vi "Save_Raw_data.vi"(4 "Add to Block Header":string, 5 "PWA Binary":i16[][](array[numeric]), 6 "Analogue Binary":i16[][](array[numeric]), 7 "append to file? (new file:F)":bool, 8 "Block Timings":T1={"Started"=0.0, "Ended"=0.0, "Analogue Frequency Hz"=1000.0} {"Analogue Frequency Hz" format="%.2f"}, 9 "LDA Binary":u16[][](array[numeric])) -> (2 "Block Header":string)   [LabVIEW 2011]
uses:
  Controls/Block_start_and_end.ctl
  Globals/LDA_meas_global_1.vi
  Globals/Constants_global.vi
  Globals/LDA_meas_global_2.vi
  Globals/Meas_global.vi
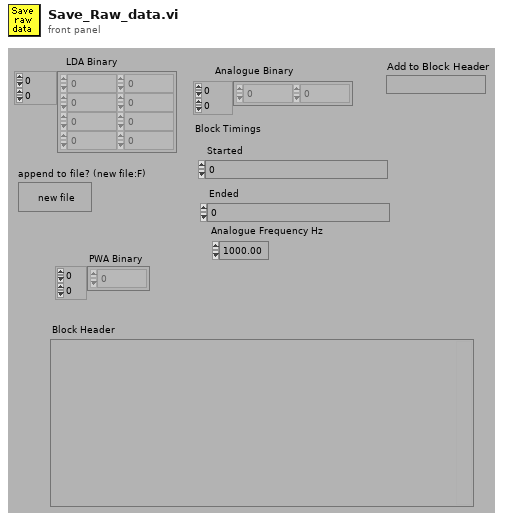
[diagram p1: front panel]
types:
  T1 = typedef "Block_start_and_end.ctl" = cluster{"Started":dbl, "Ended":dbl, "Analogue Frequency Hz":dbl}
  T2 = cluster{"scale multiplier":dbl, "scale offset":dbl}[]
  T3 = typedef "PWA_Data.ctl" = enum16{"No PWA Data", "One Ch PWA"}
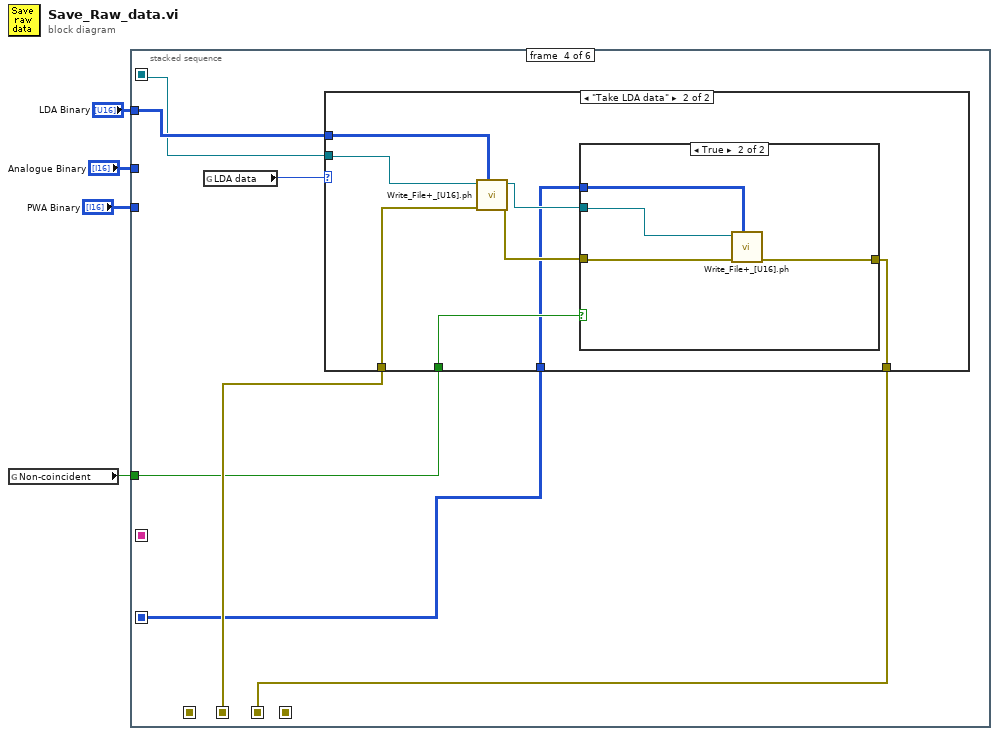
[diagram p0: block diagram]
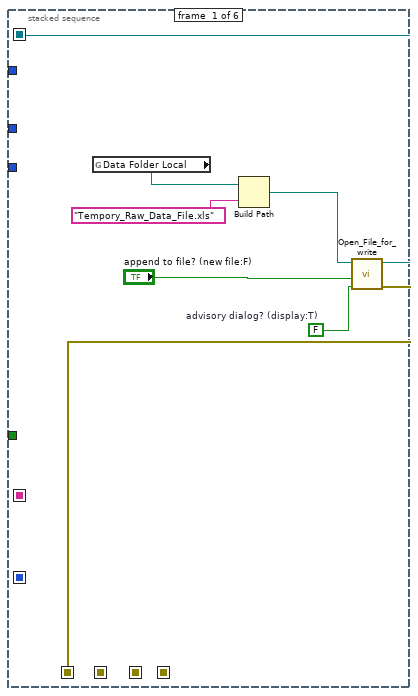
[diagram p2: hidden frame]
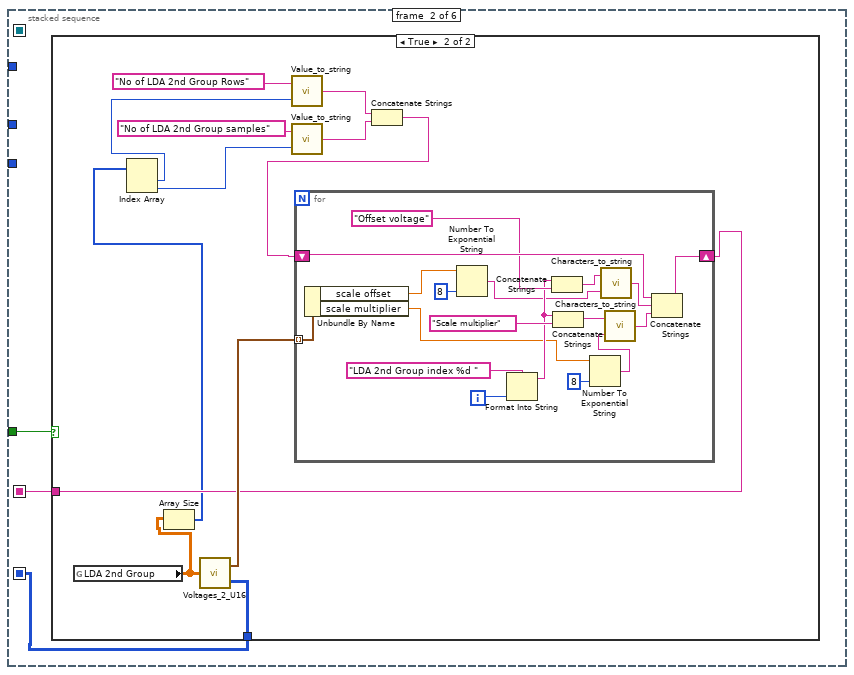
[diagram p3: hidden frame]
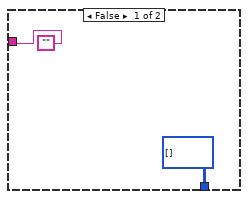
[diagram p4: hidden frame]
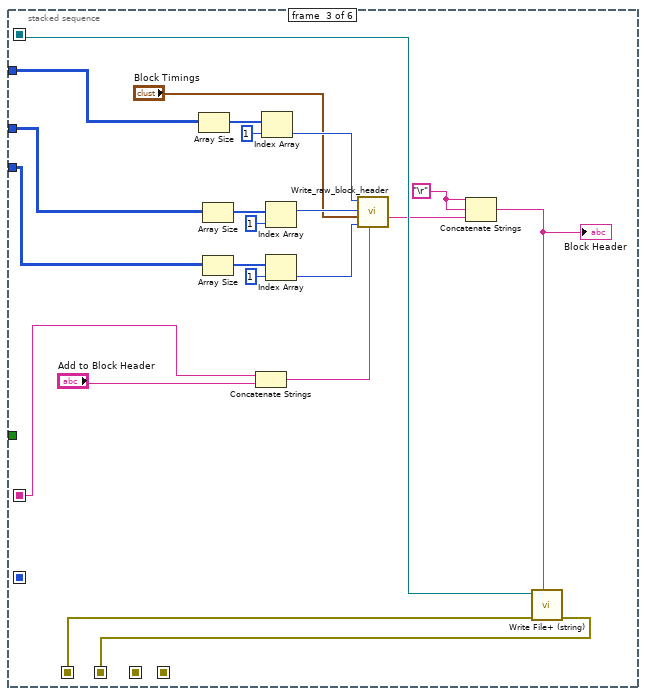
[diagram p5: hidden frame]
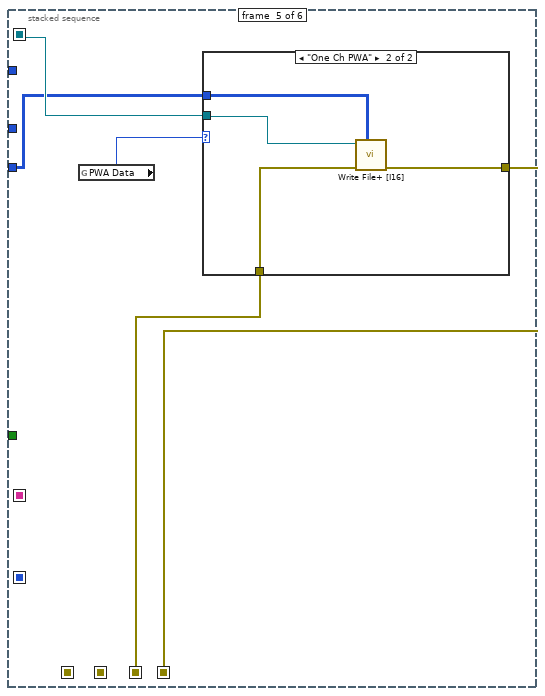
[diagram p8: hidden frame]
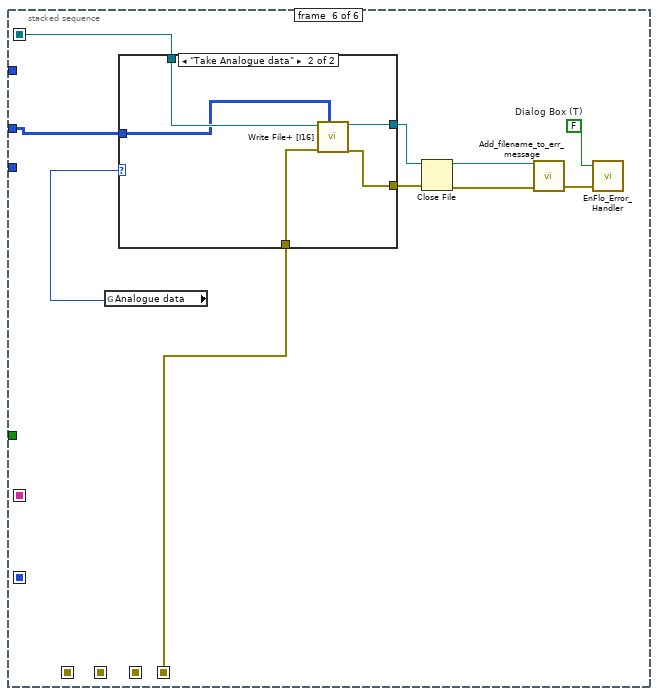
[diagram p10: hidden frame]
diagram:
  n1 = global read "LDA_meas_global_1.vi" "Non-coincident"() -> (w1:bool)
  n2 = stacked-sequence {
    seq-local: [w11 _ _ _ _ _] -> [_ _ w62 w72 w93 w108]
    seq-local: [w10 _ _ _ _ _] -> [_ _ w61 _ _ _]
    seq-local: [_ _ w60 _ _ _] -> [_ _ _ w74 _ _]
    seq-local: [_ _ _ w69 _ _] -> [_ _ _ _ w92 _]
    seq-local: [_ _ _ _ w91 _] -> [_ _ _ _ _ w100]
    seq-local: [_ w14 _ _ _ _] -> [_ _ _ w70 _ _]
    seq-local: [_ w12 _ _ _ _] -> [_ _ w48 _ _ _]
    tunnel: "LDA Binary" -> [_ _ w56 w73 _ _]
    tunnel: "Analogue Binary" -> [_ _ w55 _ _ w101]
    tunnel: "PWA Binary" -> [_ _ w52 _ w90 _]
    tunnel: w1 -> [_ w13 _ w71 _ _]
    frame #0 {
      w9 = FALSE  # advisory dialog? (display:T)
      n3 = global read "Constants_global.vi" "Data Folder Local"() -> (w8:path)
      n4 = Build Path(base path=w8, name or relative path="Tempory_Raw_Data_File.xls") -> (appended path=w6:path)
      n5 = call "Open_File_for_write.vi"("advisory dialog? (display:T)"=w9, "append to file? (new file:F)"="append to file? (new file:F)", "file path"=w6) -> ("error out"=w10:errorcluster, "refnum"=w11:refnum<file>)  [unwired: 7 out]
    }
    frame #1 {
      n6 = case shown="True" w13 {
        tunnel: [u16[][] [] ("U16 data") w28] -> w14
        tunnel: ["" w26] -> w12
        frame False {
        }
        frame True {
          n7 = global read "LDA_meas_global_2.vi" "LDA 2nd Group"() -> (w23:dbl[][])
          n8 = Array Size(array=w23) -> (size(s)=w22:i32[])
          n9 = Index Array(array=w22) -> (element #1=w21:i32, element #2=w20:i32)  [unwired: 2 in]
          n10 = call "Voltages_2_U16.vi"("Voltages"=w23) -> ("Scale and Offset"=w27:T2, "U16 data"=w28:u16[][])
          n11 = call "Value_to_string.vi"("Value"=w21, "Label for value"="No of LDA 2nd Group Rows") -> ("Output string"=w19:string)  [unwired: 1 in]
          n12 = call "Value_to_string.vi"("Value"=w20, "Label for value"="No of LDA 2nd Group samples") -> ("Output string"=w18:string)  [unwired: 1 in]
          n13 = Concatenate Strings(w19, w18) -> (w17:string)
          n14 = for {
            shift-right: [w45] -> w26
            shift-left: w17 -> [w46]
            tunnel: w27 -> [w38] mode=indexing
            i -> [w35]
            n15 = Unbundle By Name(w38) -> ("scale offset"=w31:dbl, "scale multiplier"=w34:dbl)
            n16 = Number To Exponential String(number=w31, precision (6)=i16 8) -> (E-format string=w30:string)  [unwired: 2 out]
            n17 = Format Into String(format string="LDA 2nd Group index %d ", w35) -> (resulting string=w36:string)  [unwired: 2 in, 1 out]
            n18 = Concatenate Strings(w36, "Offset voltage") -> (w33:string)
            n19 = Concatenate Strings(w36, "Scale multiplier") -> (w40:string)
            n20 = Number To Exponential String(number=w34, precision (6)=i16 8) -> (E-format string=w39:string)  [unwired: 2 out]
            n21 = call "Characters_to_string.vi"("Characters to write"=w30, "Label for characters"=w33) -> ("Output string"=w29:string)
            n22 = call "Characters_to_string.vi"("Characters to write"=w39, "Label for characters"=w40) -> ("Output string"=w41:string)
            n23 = Concatenate Strings(w46, w29, w41) -> (w45:string)
          }
        }
      }
    }
    frame #2 {
      w57 = "\r"
      n24 = Array Size(array=w56) -> (size(s)=w67:i32[])
      n25 = Array Size(array=w55) -> (size(s)=w66:i32[])
      n26 = Array Size(array=w52) -> (size(s)=w53:i32[])
      n27 = Concatenate Strings(w48, "Add to Block Header") -> (w47:string)
      n28 = Index Array(array=w67, index=1) -> (element=w64:i32)
      n29 = Index Array(array=w66, index=1) -> (element=w63:i32)
      n30 = Index Array(array=w53, index=1) -> (element=w51:i32)
      n31 = call "Write_raw_block_header.vi"("No of LDA samples"=w64, "No of analogue samples"=w63, "Block Timings"="Block Timings", "No of PWA samples"=w51, "Add to Block Header"=w47) -> ("Output string"=w58:string)
      n32 = Concatenate Strings(w57, w57, w58) -> (w50:string)
      "Block Header" <- w50
      n33 = call <vilib>:"Write File+ (string).vi"("string"=w50, "error in (no error)"=w61, "refnum"=w62) -> ("error out"=w60:errorcluster)  [unwired: 2 in, 4 out]
    }
    frame #3 {
      n34 = global read "Meas_global.vi" "LDA data"() -> (w75:enum16{"No LDA data", "Take LDA data"})
      n35 = case shown="\"Take LDA data\"" w75 {
        tunnel: w73 -> [_ w84]
        tunnel: w72 -> [_ w83]
        tunnel: w74 -> [w76 w82]
        tunnel: w71 -> [_ w81]
        tunnel: w70 -> [_ w77]
        tunnel: [w76 w78] -> w69
        frame "No LDA data" {
        }
        frame "Take LDA data" {
          n36 = call "Write_File+_[U16].ph.vi"("2D array"=w84, "error in (no error)"=w82, "refnum"=w83) -> ("error out"=w79:errorcluster, "dup refnum"=w80:refnum<file>)  [unwired: 3 in, 4 out]
          n37 = case shown="True" w81 {
            tunnel: w77 -> [_ w89]
            tunnel: w80 -> [_ w88]
            tunnel: [w85 w87] -> w78
            tunnel: w79 -> [w85 w86]
            frame False {
            }
            frame True {
              n38 = call "Write_File+_[U16].ph.vi"("2D array"=w89, "error in (no error)"=w86, "refnum"=w88) -> ("error out"=w87:errorcluster)  [unwired: 3 in, 5 out]
            }
          }
        }
      }
    }
    frame #4 {
      n39 = global read "Meas_global.vi" "PWA Data"() -> (w94:T3)
      n40 = case shown="\"One Ch PWA\"" w94 {
        tunnel: w90 -> [_ w97]
        tunnel: w93 -> [_ w96]
        tunnel: w92 -> [w95 w99]
        tunnel: [w95 w98] -> w91
        frame "No PWA Data" {
        }
        frame "One Ch PWA" {
          n41 = call <vilib>:"Write File+ [I16].vi"("2D array"=w97, "error in (no error)"=w99, "refnum"=w96) -> ("error out"=w98:errorcluster)  [unwired: 3 in, 5 out]
        }
      }
    }
    frame #5 {
      w106 = FALSE  # Dialog Box (T)
      n42 = global read "Meas_global.vi" "Analogue data"() -> (w109:enum16{"No Analogue data", "Take Analogue data"})
      n43 = case shown="\"Take Analogue data\"" w109 {
        tunnel: w101 -> [_ w115]
        tunnel: w108 -> [w111 w116]
        tunnel: w100 -> [w110 w114]
        tunnel: [w110 w113] -> w105
        tunnel: [w111 w112] -> w104
        frame "No Analogue data" {
        }
        frame "Take Analogue data" {
          n44 = call <vilib>:"Write File+ [I16].vi"("2D array"=w115, "error in (no error)"=w114, "refnum"=w116) -> ("error out"=w113:errorcluster, "dup refnum"=w112:refnum<file>)  [unwired: 3 in, 4 out]
        }
      }
      n45 = Close File(refnum=w104, error in=w105) -> (path=w102:path, error out=w103:errorcluster)
      n46 = call "Add_filename_to_err_message.vi"("error in (no error)"=w103, "Path"=w102) -> ("error out"=w107:errorcluster)
      n47 = call "EnFlo_Error_Handler.vi"("error in (no error)"=w107, "Dialog Box (T)"=w106) -> ()  [unwired: 1 in, 3 out]
    }
  }
